vi "Find Devices (uSMC).vi"(8 "error in (no error)":errorcluster) -> (0 "error out":errorcluster, 1 "Number of Devices Found":i32, 3 "Visa array out":refnum<visa-resource-name>[](array[refnum]))   [LabVIEW 2010, in "SignalWriterMH110203USBStepperMotor.lvclass"]
uses:
  SignalWriterMH110203USBStepperMotor.lvclass
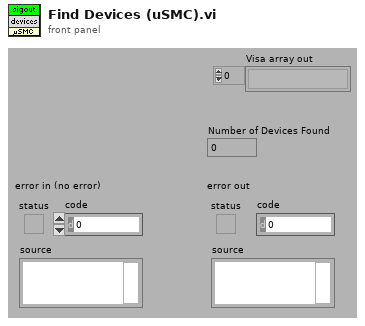
[diagram p1: front panel]
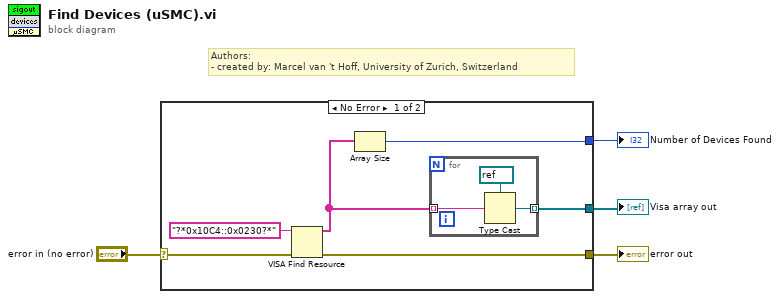
[diagram p0: block diagram]
diagram:
  # "Authors: \n- created by: Marcel van 't Hoff, University of Zurich, Switzerland"
  n1 = case shown="No Error" "error in (no error)" {
    selector: "error in (no error)" -> [w7 w14]
    tunnel: [w5 _] -> w4
    tunnel: [w9 w14] -> w3
    tunnel: [w8 _] -> w2
    frame No Error {
      n2 = VISA Find Resource(8:w7, 11:"?*0x10C4::0x0230?*" ("expression (\"?*\")")) -> (0:w9:errorcluster, 3:w6:string[])  [unwired: 1 in, 1 out]
      n3 = Array Size(array=w6) -> (size(s)=w8:i32)
      n4 = for {
        tunnel: w6 -> [w13] mode=indexing
        tunnel: [w11] -> w5 mode=indexing
        n5 = Type Cast(type=refnum<visa-resource-name> refnum ("VISA resource name"), x=w13) -> (*(type *) &x=w11:refnum<visa-resource-name>)
      }
    }
    frame Error {
    }
  }
  "error out" <- w3
  "Visa array out" <- w4
  "Number of Devices Found" <- w2
